vi "Global.vi"() -> ()   [LabVIEW 2017]
uses:
  <vilib>/addons/database/Connection.llb/Conn ObjectReference.ctl
  <vilib>/addons/database/NI_Database_API.lvlib
panel:
  in  "Database Ref":T1
  in  "Proyectos Path":path=path "\\\\DLINK-E74F4C\\ALT Pub/ALT Contabilizador/Proyectos.txt"
  in  "User Path":path=path "\\\\DLINK-E74F4C\\ALT Pub/ALT Contabilizador/users.cfg"
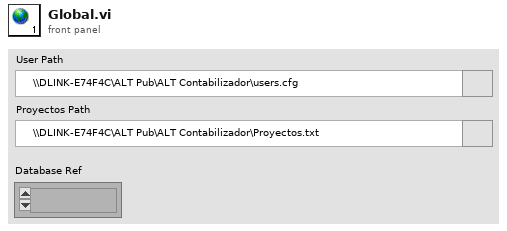
[diagram p1: front panel]
types:
  T1 = typedef "NI_Database_API.lvlib/Conn ObjectReference.ctl" = refnum<k1>
diagram:
